vi "CAL-Load data.vi"(0 "user path":path, 9 "Desired Fs (Hz)":dbl, 11 "error in (no error)":errorcluster) -> (3 "Smooth Params":T1={"Method"=enum."Loess", "MA"={"Iterations"=100, "Length"=3}, "Loess"={"Length"=21, "Type"=enum."Quadratic", "Robust"=TRUE}} {"Loess"."Length" min=1 step=1; "MA"."Length" min=1 step=1; "MA"."Iterations" min=1 step=1}, 4 "Frequency (Hz)":dbl[](array[numeric]), 6 "Mag":dbl[](array[numeric]), 8 "Phase":dbl[](array[numeric]), 10 "Unsmoothed Mag":dbl[](array[numeric]), 13 "npts":i32, 14 "Fs (Hz)":dbl, 15 "error out":errorcluster)   [LabVIEW 2020]
uses:
  In-Ear Calibration VIs/LV Source/Type Defs/Cal-Smoothing Parameters.ctl
  epl-vi-lib/Utility VIs/Array Manipulation VIs/Array-Dimensions (2D).vi
  epl-vi-lib/Utility VIs/Array Manipulation VIs/Irregular Array Subset (DBL).vi
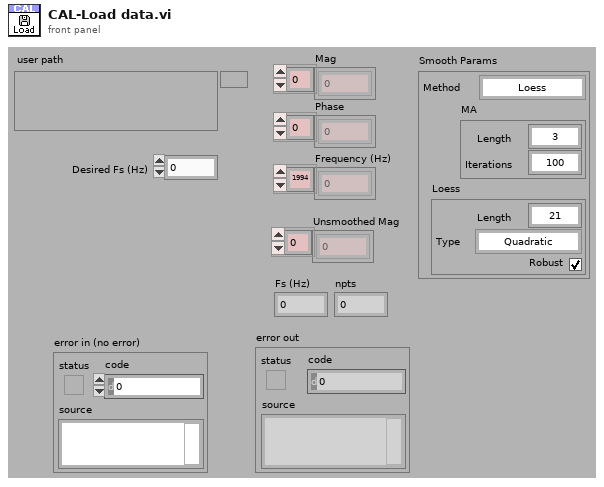
[diagram p1: front panel]
types:
  T1 = typedef "Cal-Smoothing Parameters.ctl" = cluster{"Method":enum16{"None", "Moving average", "Loess"}, "MA":cluster{"Iterations":i32, "Length":i32}, "Loess":cluster{"Length":i32, "Type":enum16{"Linear", "Quadratic"}, "Robust":bool}}
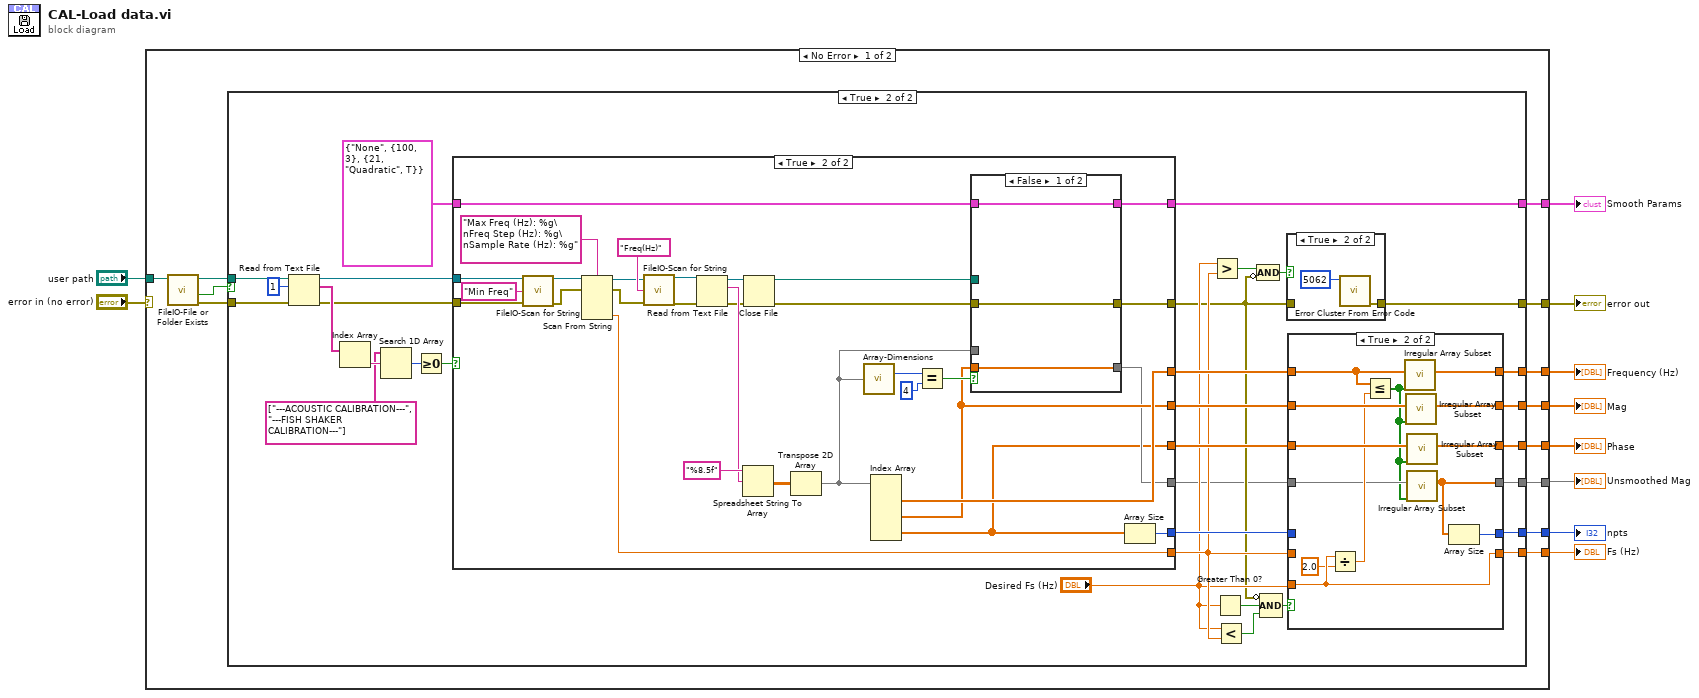
[diagram p0: block diagram]
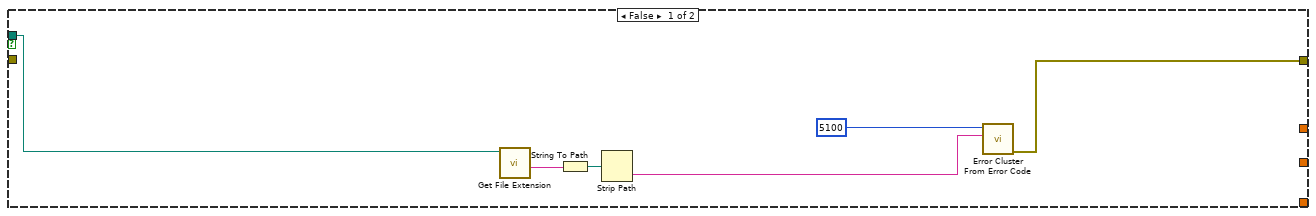
[diagram p2: hidden frame]
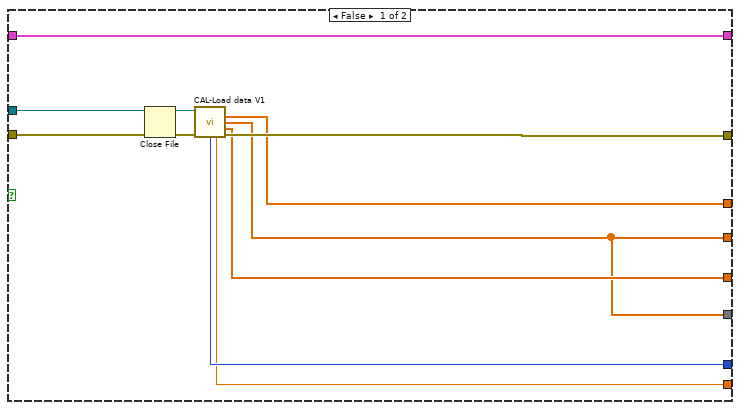
[diagram p5: hidden frame]
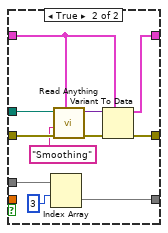
[diagram p6: hidden frame]
diagram:
  n1 = case shown="No Error" "error in (no error)" {
    selector: "error in (no error)" -> [_ w139]
    tunnel: "user path" -> [w18 _]
    tunnel: [w19 w139] -> w8
    tunnel: [w17 _] -> w7
    tunnel: [w16 _] -> w6
    tunnel: [w15 _] -> w5
    tunnel: [w14 _] -> w4
    tunnel: [w13 _] -> w3
    tunnel: [w12 _] -> w2
    tunnel: [w11 _] -> w1
    frame No Error {
      n2 = call "FileIO-File or Folder Exists.vi"("path"=w18) -> ("error out"=w21:errorcluster, "Exists?"=w20:bool, "dup path"=w22:path)  [unwired: 7 in, 1 out]
      n3 = case shown="True" w20 {
        tunnel: w22 -> [w26 w60]
        tunnel: w21 -> [_ w59]
        tunnel: [w27 w52] -> w19
        tunnel: [_ w40] -> w17
        tunnel: [_ w39] -> w16
        tunnel: [_ w38] -> w15
        tunnel: [_ w37] -> w14
        tunnel: [_ w36] -> w13
        tunnel: [_ w34] -> w12
        tunnel: [_ w32] -> w11
        frame False {
          n4 = call <vilib>:"Get File Extension.vi"("file"=w26) -> ("filename without extension"=w24:string)  [unwired: 6 in, 4 out]
          n5 = String To Path(string=w24) -> (path=w25:path)
          n6 = Strip Path(path=w25) -> (name=w23:string)  [unwired: 1 out]
          n7 = call <vilib>:"Error Cluster From Error Code.vi"("error message (\"\")"=w23, "error code (0)"=5100) -> ("error out"=w27:errorcluster)  [unwired: 7 in]
        }
        frame True {
          n8 = Read from Text File(file (use dialog)=w60, count=1, error in=w59) -> (refnum out=w55:refnum<file>, text=w57:string[], error out=w54:errorcluster)  [unwired: 1 in, 1 out]
          n9 = Index Array(array=w57) -> (element=w31:string)  [unwired: 1 in]
          n10 = Search 1D Array(1D array=string[] ["---ACOUSTIC CALIBRATION---", "---FISH SHAKER CALIBRATION---"], element=w31) -> (index of element=w29:i32)  [unwired: 1 in]
          n11 = Greater Or Equal To 0?(x=w29) -> (x >= 0?=w56:bool)
          n12 = case shown="True" w56 {
            tunnel: w55 -> [w92 w118]
            tunnel: w54 -> [w93 w117]
            tunnel: [w87 w121] -> w50
            tunnel: [w89 w97] -> w41
            tunnel: [w84 w102] -> w49
            tunnel: [w88 w99] -> w48
            tunnel: [w85 w113] -> w46
            tunnel: [w86 w100] -> w47
            tunnel: [w84 w101] -> w35
            tunnel: T1 {"Method"=enum."None", "MA"={"Iterations"=100, "Length"=3}, "Loess"={"Length"=21, "Type"=enum."Quadratic", "Robust"=TRUE}} ("Smooth Params") -> [w83 w95]
            tunnel: [w83 w94] -> w32
            frame False {
              n13 = Close File(refnum=w92, error in=w93) -> (path=w91:path, error out=w90:errorcluster)
              n14 = call "CAL-Load data V1.vi"("user path"=w91, "error in (no error)"=w90) -> ("Frequency"=w87:dbl[], "Mag"=w84:dbl[], "Phase"=w88:dbl[], "npts"=w86:i32, "Fs (Hz)"=w85:dbl, "error out"=w89:errorcluster)  [unwired: 7 in, 1 out]
            }
            frame True {
              n15 = call "FileIO-Scan for String.vi"("File Refnum"=w118, "regular expression"="Min Freq", "error IO"=w117) -> ("refnum out"=w115:refnum<file>, "error out"=w116:errorcluster)  [unwired: 9 in, 2 out]
              n16 = Scan From String("Max Freq (Hz): %g\nFreq Step (Hz): %g\nSample Rate (Hz): %g", w115, w116) -> (w110:refnum<file>, w111:errorcluster, output 3=w113:dbl)  [unwired: 5 in]
              n17 = call "FileIO-Scan for String.vi"("File Refnum"=w110, "regular expression"="Freq(Hz)", "error IO"=w111) -> ("refnum out"=w109:refnum<file>, "error out"=w108:errorcluster)  [unwired: 9 in, 2 out]
              n18 = Read from Text File(file (use dialog)=w109, error in=w108) -> (refnum out=w120:refnum<file>, text=w122:string, error out=w119:errorcluster)  [unwired: 2 in, 1 out]
              n19 = Spreadsheet String To Array(format string="%8.5f" ("format (%.3f)"), spreadsheet string=w122) -> (array=w105:dbl[][])  [unwired: 2 in]
              n20 = Close File(refnum=w120, error in=w119) -> (path=w96:path, error out=w98:errorcluster)
              n21 = Transpose 2D Array(2D array=w105) -> (transposed array=w104:dbl[][])
              n22 = call-poly "Array-Dimensions.vi"("2D Array"=w104) -> ("# rows"=w103:i32)  [unwired: 13 in, 1 out]
              n23 = Index Array(array=w104) -> (element #1=w121:dbl[], element #2=w102:dbl[], element #3=w99:dbl[])  [unwired: 6 in]
              n24 = Equal?(x=w103, y=4) -> (x = y?=w106:bool)
              n25 = case shown="False" w106 {
                tunnel: w104 -> [_ w138]
                tunnel: w102 -> [w127 _]
                tunnel: [w127 w136] -> w101
                tunnel: w98 -> [w126 w135]
                tunnel: [w126 w130] -> w97
                tunnel: w96 -> [_ w133]
                tunnel: w95 -> [w125 w129]
                tunnel: [w125 w128] -> w94
                frame False {
                }
                frame True {
                  n26 = Index Array(array=w138, index (row)=3) -> (element=w136:dbl[])  [unwired: 1 in]
                  n27 = call "Read Anything.vi"("Type of Anything"=w129, "Error In"=w135, "Section Name (Name of \"Type of Anything\")"="Smoothing" ("Section Name (Name of \"Type of Anything\")"), "Path (dialog)"=w133) -> ("Error Out"=w132:errorcluster, "Anything"=w131:variant)  [unwired: 5 in, 1 out]
                  n28 = Variant To Data(error in=w132, type=w129, Variant=w131) -> (data=w128:T1, error out=w130:errorcluster)
                }
              }
              n29 = Array Size(array=w99) -> (size(s)=w100:i32)
            }
          }
          n30 = Greater?(x="Desired Fs (Hz)", y=w46) -> (0:w53:bool)
          n31 = Greater Than 0?(x="Desired Fs (Hz)") -> (x > 0?=w44:bool)
          n32 = Less?(x="Desired Fs (Hz)", y=w46) -> (x < y?=w45:bool)
          n33 = Compound Arithmetic op=AND(w53, invert w41) -> (w51:bool)
          n34 = Compound Arithmetic op=AND(invert w41, w44, w45) -> (w43:bool)
          n35 = case shown="True" w51 {
            tunnel: w41 -> [w80 _]
            tunnel: [w80 w82] -> w52
            frame False {
            }
            frame True {
              n36 = call <vilib>:"Error Cluster From Error Code.vi"("error code (0)"=5062) -> ("error out"=w82:errorcluster)  [unwired: 8 in]
            }
          }
          n37 = case shown="True" w43 {
            tunnel: w50 -> [w66 w77]
            tunnel: w49 -> [w65 w78]
            tunnel: w48 -> [w64 w75]
            tunnel: w47 -> [w63 _]
            tunnel: [w66 w79] -> w40
            tunnel: [w65 w76] -> w39
            tunnel: [w64 w73] -> w38
            tunnel: [w63 w74] -> w37
            tunnel: [w62 w72] -> w36
            tunnel: w46 -> [w62 _]
            tunnel: "Desired Fs (Hz)" -> [_ w72]
            tunnel: w35 -> [w61 w69]
            tunnel: [w61 w67] -> w34
            frame False {
            }
            frame True {
              n38 = Divide(x=w72, y=2.0) -> (x/y=w71:dbl)
              n39 = Less Or Equal?(x=w77, y=w71) -> (x <= y?=w68:bool[])
              n40 = call-poly "Irregular Array Subset.vi"("Mask"=w68, "Array"=w77) -> ("Array Subset"=w79:dbl[])  [unwired: 8 in, 1 out]
              n41 = call-poly "Irregular Array Subset.vi"("Mask"=w68, "Array"=w78) -> ("Array Subset"=w76:dbl[])  [unwired: 8 in, 1 out]
              n42 = call-poly "Irregular Array Subset.vi"("Mask"=w68, "Array"=w75) -> ("Array Subset"=w73:dbl[])  [unwired: 8 in, 1 out]
              n43 = call-poly "Irregular Array Subset.vi"("Mask"=w68, "Array"=w69) -> ("Array Subset"=w67:dbl[])  [unwired: 8 in, 1 out]
              n44 = Array Size(array=w67) -> (size(s)=w74:i32)
            }
          }
        }
      }
    }
    frame Error {
    }
  }
  "error out" <- w8
  "Smooth Params" <- w1
  "Frequency (Hz)" <- w7
  "Mag" <- w6
  "Phase" <- w5
  "Fs (Hz)" <- w3
  "npts" <- w4
  "Unsmoothed Mag" <- w2
